vi "FeedbackDecode_UpdateDecodeClustElect.vi"(2 "DecodeClustIn":T1={"TrainParams"={"Lag"=0.0, "KernelWidth"=0.3, "TargRad"=0.15}, "Kinematics"={"Thumb"=0.0, "Index"=0.0, "Middle"=0.0, "Ring"=0.0, "Little"=0.0, "ThumbInt"=0.0, "IndexInt"=0.0, "RingInt"=0.0, "LittleInt"=0.0, "Wrist"=0.0, "WristYaw"=0.0, "WristRoll"=0.0}, "CtrlButtons"={"AcqTraining"=FALSE, "ApplyBaseline"=FALSE, "ApplyTraining"=FALSE, "LoadTrainFile"=FALSE, "CAR"=FALSE, "NIPSpikes"=FALSE, "AcqBaseline"=FALSE, "Stop"=FALSE, "ResetTrial"=FALSE, "CalDEKA"=FALSE, "HideSphrs"=FALSE, "StartTrials"=FALSE, "AutoPop"=FALSE, "ResetVRE"=FALSE, "StopVRE"=FALSE, "AcqCAR"=FALSE, "ConARD"=FALSE, "DEKARestart"=FALSE, "ConnDEKA"=FALSE}, "CompID"={"LV"={"Name"="PNILABVIEW", "IP"="155.100.90.215"}, "ML"={"Name"="PNIMATLAB", "IP"="155.100.91.231"}}, "KMvntClust"={"KGain"=[[1.0, 1.0, -1.0, 1.0], [1.0, 1.0, -1.0, 1.0], [1.0, 1.0, -1.0, 1.0], [1.0, 1.0, -1.0, 1.0], [1.0, 1.0, -1.0, 1.0], [1.0, 1.0, -1.0, 1.0], [1.0, 1.0, -1.0, 1.0], [1.0, 1.0, -1.0, 1.0], [1.0, 1.0, -1.0, 1.0], [1.0, 1.0, -1.0, 1.0], [1.0, 1.0, -1.0, 1.0], [1.0, 1.0, -1.0, 1.0]], "KMvnts"={"Thumb"=FALSE, "Index"=FALSE, "Middle"=FALSE, "Ring"=FALSE, "Little"=FALSE, "ThumbInt"=FALSE, "IndexInt"=FALSE, "RingInt"=FALSE, "LittleInt"=FALSE, "WristPitch"=FALSE, "WristYaw"=FALSE, "WristRoll"=FALSE}, "KThresh"=[[0.2, 0.2, -1.0, 1.0], [0.2, 0.2, -1.0, 1.0], [0.2, 0.2, -1.0, 1.0], [0.2, 0.2, -1.0, 1.0], [0.2, 0.2, -1.0, 1.0], [0.2, 0.2, -1.0, 1.0], [0.2, 0.2, -1.0, 1.0], [0.2, 0.2, -1.0, 1.0], [0.2, 0.2, -1.0, 1.0], [0.2, 0.2, -1.0, 1.0], [0.2, 0.2, -1.0, 1.0], [0.2, 0.2, -1.0, 1.0]], "CtrlMode"=[], "CtrlSpd"=[]}, "ClearUEA"=FALSE, "Targets"={"Thumb"=0.0, "Index"=0.0, "Middle"=0.0, "Ring"=0.0, "Little"=0.0, "ThumbInt"=0.0, "IndexInt"=0.0, "RingInt"=0.0, "LittleInt"=0.0, "Wrist"=0.0, "WristYaw"=0.0, "WristRoll"=0.0}, "KUEAArray"=[{"Boolean 1"=FALSE, "Boolean 2"=FALSE, "Boolean 3"=FALSE, "Boolean 4"=FALSE, "Boolean 5"=FALSE, "Boolean 6"=FALSE, "Boolean 7"=FALSE, "Boolean 8"=FALSE, "Boolean 9"=FALSE, "Boolean 10"=FALSE, "Boolean 11"=FALSE, "Boolean 12"=FALSE, "Boolean 13"=FALSE, "Boolean 14"=FALSE, "Boolean 15"=FALSE, "Boolean 16"=FALSE, "Boolean 17"=FALSE, "Boolean 18"=FALSE, "Boolean 19"=FALSE, "Boolean 20"=FALSE, "Boolean 21"=FALSE, "Boolean 22"=FALSE, "Boolean 23"=FALSE, "Boolean 24"=FALSE, "Boolean 25"=FALSE, "Boolean 26"=FALSE, "Boolean 27"=FALSE, "Boolean 28"=FALSE, "Boolean 29"=FALSE, "Boolean 30"=FALSE, "Boolean 31"=FALSE, "Boolean 32"=FALSE, "Boolean 33"=FALSE, "Boolean 34"=FALSE, "Boolean 35"=FALSE, "Boolean 36"=FALSE, "Boolean 37"=FALSE, "Boolean 38"=FALSE, "Boolean 39"=FALSE, "Boolean 40"=FALSE, "Boolean 41"=FALSE, "Boolean 42"=FALSE, "Boolean 43"=FALSE, "Boolean 44"=FALSE, "Boolean 45"=FALSE, "Boolean 46"=FALSE, "Boolean 47"=FALSE, "Boolean 48"=FALSE, "Boolean 49"=FALSE, "Boolean 50"=FALSE, "Boolean 51"=FALSE, "Boolean 52"=FALSE, "Boolean 53"=FALSE, "Boolean 54"=FALSE, "Boolean 55"=FALSE, "Boolean 56"=FALSE, "Boolean 57"=FALSE, "Boolean 58"=FALSE, "Boolean 59"=FALSE, "Boolean 60"=FALSE, "Boolean 61"=FALSE, "Boolean 62"=FALSE, "Boolean 63"=FALSE, "Boolean 64"=FALSE, "Boolean 65"=FALSE, "Boolean 66"=FALSE, "Boolean 67"=FALSE, "Boolean 68"=FALSE, "Boolean 69"=FALSE, "Boolean 70"=FALSE, "Boolean 71"=FALSE, "Boolean 72"=FALSE, "Boolean 73"=FALSE, "Boolean 74"=FALSE, "Boolean 75"=FALSE, "Boolean 76"=FALSE, "Boolean 77"=FALSE, "Boolean 78"=FALSE, "Boolean 79"=FALSE, "Boolean 80"=FALSE, "Boolean 81"=FALSE, "Boolean 82"=FALSE, "Boolean 83"=FALSE, "Boolean 84"=FALSE, "Boolean 85"=FALSE, "Boolean 86"=FALSE, "Boolean 87"=FALSE, "Boolean 88"=FALSE, "Boolean 89"=FALSE, "Boolean 90"=FALSE, "Boolean 91"=FALSE, "Boolean 92"=FALSE, "Boolean 93"=FALSE, "Boolean 94"=FALSE, "Boolean 95"=FALSE, "Boolean 96"=FALSE, "Boolean 97"=FALSE, "Boolean 98"=FALSE, "Boolean 99"=FALSE, "Boolean 100"=FALSE}, {"Boolean 1"=FALSE, "Boolean 2"=FALSE, "Boolean 3"=FALSE, "Boolean 4"=FALSE, "Boolean 5"=FALSE, "Boolean 6"=FALSE, "Boolean 7"=FALSE, "Boolean 8"=FALSE, "Boolean 9"=FALSE, "Boolean 10"=FALSE, "Boolean 11"=FALSE, "Boolean 12"=FALSE, "Boolean 13"=FALSE, "Boolean 14"=FALSE, "Boolean 15"=FALSE, "Boolean 16"=FALSE, "Boolean 17"=FALSE, "Boolean 18"=FALSE, "Boolean 19"=FALSE, "Boolean 20"=FALSE, "Boolean 21"=FALSE, "Boolean 22"=FALSE, "Boolean 23"=FALSE, "Boolean 24"=FALSE, "Boolean 25"=FALSE, "Boolean 26"=FALSE, "Boolean 27"=FALSE, "Boolean 28"=FALSE, "Boolean 29"=FALSE, "Boolean 30"=FALSE, "Boolean 31"=FALSE, "Boolean 32"=FALSE, "Boolean 33"=FALSE, "Boolean 34"=FALSE, "Boolean 35"=FALSE, "Boolean 36"=FALSE, "Boolean 37"=FALSE, "Boolean 38"=FALSE, "Boolean 39"=FALSE, "Boolean 40"=FALSE, "Boolean 41"=FALSE, "Boolean 42"=FALSE, "Boolean 43"=FALSE, "Boolean 44"=FALSE, "Boolean 45"=FALSE, "Boolean 46"=FALSE, "Boolean 47"=FALSE, "Boolean 48"=FALSE, "Boolean 49"=FALSE, "Boolean 50"=FALSE, "Boolean 51"=FALSE, "Boolean 52"=FALSE, "Boolean 53"=FALSE, "Boolean 54"=FALSE, "Boolean 55"=FALSE, "Boolean 56"=FALSE, "Boolean 57"=FALSE, "Boolean 58"=FALSE, "Boolean 59"=FALSE, "Boolean 60"=FALSE, "Boolean 61"=FALSE, "Boolean 62"=FALSE, "Boolean 63"=FALSE, "Boolean 64"=FALSE, "Boolean 65"=FALSE, "Boolean 66"=FALSE, "Boolean 67"=FALSE, "Boolean 68"=FALSE, "Boolean 69"=FALSE, "Boolean 70"=FALSE, "Boolean 71"=FALSE, "Boolean 72"=FALSE, "Boolean 73"=FALSE, "Boolean 74"=FALSE, "Boolean 75"=FALSE, "Boolean 76"=FALSE, "Boolean 77"=FALSE, "Boolean 78"=FALSE, "Boolean 79"=FALSE, "Boolean 80"=FALSE, "Boolean 81"=FALSE, "Boolean 82"=FALSE, "Boolean 83"=FALSE, "Boolean 84"=FALSE, "Boolean 85"=FALSE, "Boolean 86"=FALSE, "Boolean 87"=FALSE, "Boolean 88"=FALSE, "Boolean 89"=FALSE, "Boolean 90"=FALSE, "Boolean 91"=FALSE, "Boolean 92"=FALSE, "Boolean 93"=FALSE, "Boolean 94"=FALSE, "Boolean 95"=FALSE, "Boolean 96"=FALSE, "Boolean 97"=FALSE, "Boolean 98"=FALSE, "Boolean 99"=FALSE, "Boolean 100"=FALSE}], "ReTrain"=FALSE, "TargDist"=[0.0, 0.0, 0.0, 0.0, 0.0, 0.0], "State"=enum."Initialize", "KalmanType"=enum."Standard", "EventStr"="", "SelElect"=1.0, "KinSrc"=enum."Training", "HoverElect"=0.0, "RasterWin"=1.0, "WfCnt"=15.0, "ClearWfs"=FALSE, "ApplyThresh"=FALSE, "ThreshVal"=-5.0, "ThreshMode"=enum."RMS Single", "DataFolder"="00000000-000000", "ClearEMG"=FALSE, "KEMGClust"={"Boolean 92"=FALSE, "Boolean 82"=FALSE, "Boolean 72"=FALSE, "Boolean 62"=FALSE, "Boolean 52"=FALSE, "Boolean 42"=FALSE, "Boolean 32"=FALSE, "Boolean 22"=FALSE, "Boolean 12"=FALSE, "Boolean 2"=FALSE, "Boolean 93"=FALSE, "Boolean 83"=FALSE, "Boolean 73"=FALSE, "Boolean 63"=FALSE, "Boolean 53"=FALSE, "Boolean 43"=FALSE, "Boolean 33"=FALSE, "Boolean 23"=FALSE, "Boolean 13"=FALSE, "Boolean 3"=FALSE, "Boolean 94"=FALSE, "Boolean 84"=FALSE, "Boolean 74"=FALSE, "Boolean 64"=FALSE, "Boolean 54"=FALSE, "Boolean 44"=FALSE, "Boolean 34"=FALSE, "Boolean 24"=FALSE, "Boolean 14"=FALSE, "Boolean 4"=FALSE, "Boolean 95"=FALSE, "Boolean 85"=FALSE, "Boolean 75"=FALSE, "Boolean 65"=FALSE, "Boolean 55"=FALSE, "Boolean 45"=FALSE, "Boolean 35"=FALSE, "Boolean 25"=FALSE, "Boolean 15"=FALSE, "Boolean 5"=FALSE, "Boolean 96"=FALSE, "Boolean 86"=FALSE, "Boolean 76"=FALSE, "Boolean 66"=FALSE, "Boolean 56"=FALSE, "Boolean 46"=FALSE, "Boolean 36"=FALSE, "Boolean 26"=FALSE, "Boolean 16"=FALSE, "Boolean 6"=FALSE, "Boolean 97"=FALSE, "Boolean 87"=FALSE, "Boolean 77"=FALSE, "Boolean 67"=FALSE, "Boolean 57"=FALSE, "Boolean 47"=FALSE, "Boolean 37"=FALSE, "Boolean 27"=FALSE, "Boolean 17"=FALSE, "Boolean 7"=FALSE, "Boolean 98"=FALSE, "Boolean 88"=FALSE, "Boolean 78"=FALSE, "Boolean 68"=FALSE, "Boolean 58"=FALSE, "Boolean 48"=FALSE, "Boolean 38"=FALSE, "Boolean 28"=FALSE, "Boolean 18"=FALSE, "Boolean 8"=FALSE, "Boolean 99"=FALSE, "Boolean 89"=FALSE, "Boolean 79"=FALSE, "Boolean 69"=FALSE, "Boolean 59"=FALSE, "Boolean 49"=FALSE, "Boolean 39"=FALSE, "Boolean 29"=FALSE, "Boolean 19"=FALSE, "Boolean 9"=FALSE}, "EvntFlag"=FALSE, "FillUEA"=FALSE, "FillEMG"=FALSE, "FillMvnts"=FALSE, "BadUEAElects"=[], "KEMGExtra"=[], "AllPairs"=FALSE, "AutoThresh"=0.4, "BadEMGChans"=[], "LinkedDOF"="{}", "AutoPopType"=enum."Standard", "CARType"=enum."Standard", "*Map"=enum."pNeural/pEMG", "GainFill"=1.0, "ThreshFill"=1.0, "TestType"=enum."MSMS", "Outcome"=enum."---", "TrialCnt"=[], "ClearTrials"=FALSE, "Log10"=FALSE, "KDFFile"="{}", "LimitExt"=FALSE, "*Prosthesis"=enum."MaleLeft", "StartML"=FALSE, "StartMLAux"=FALSE, "StartRec"=FALSE, "DynaThr"=FALSE, "ModeFill"=enum."Position", "SpdFill"=1.0, "DEKAMode"=enum."Velocity", "FreeParam"=0.4, "GoalNoise"=0.4, "Load NN"=FALSE, "ExportTrain"=FALSE, "NumComp"=enum."2 Computers", "DataDir"="00000000-000000", "BuildDir"="00000000-000000", "LatchingFilter"=FALSE, "Trigger"=FALSE, "StartARD"=FALSE, "StartTaska"=FALSE, "StartTaskaSens"=FALSE, "BarBtn"=FALSE} {"SpdFill" min=0.0 max=10.0 step=0.1; "RasterWin" min=1.0 max=30.0 step=1.0; "ThreshFill" min=0.0 max=10.0 step=0.01; "GainFill" min=0.0 max=10.0 step=0.1; "AutoThresh" min=0.0 max=1.0; "Targets"."LittleInt" min=0.0 max=1.0 step=0.01; "Targets"."WristRoll" min=0.0 max=1.0 step=0.01; "Targets"."WristYaw" min=0.0 max=1.0 step=0.01; "Targets"."Wrist" min=0.0 max=1.0 step=0.01; "Targets"."Little" min=0.0 max=1.0 step=0.01; "Targets"."Thumb" min=0.0 max=1.0 step=0.01; "Targets"."RingInt" min=0.0 max=1.0 step=0.01; "Targets"."IndexInt" min=0.0 max=1.0 step=0.01; "Targets"."ThumbInt" min=0.0 max=1.0 step=0.01; "Targets"."Ring" min=0.0 max=1.0 step=0.01; "Targets"."Middle" min=0.0 max=1.0 step=0.01; "Targets"."Index" min=0.0 max=1.0 step=0.01; "KMvntClust"."CtrlSpd" min=0 max=10; "KMvntClust"."KThresh" min=0 max=1; "KMvntClust"."KGain" min=0; "Kinematics"."LittleInt" min=0.0 max=1.0 step=0.01; "Kinematics"."WristRoll" min=0.0 max=1.0 step=0.01; "Kinematics"."WristYaw" min=0.0 max=1.0 step=0.01; "Kinematics"."Wrist" min=0.0 max=1.0 step=0.01; "Kinematics"."Little" min=0.0 max=1.0 step=0.01; "Kinematics"."Thumb" min=0.0 max=1.0 step=0.01; "Kinematics"."RingInt" min=0.0 max=1.0 step=0.01; "Kinematics"."IndexInt" min=0.0 max=1.0 step=0.01; "Kinematics"."ThumbInt" min=0.0 max=1.0 step=0.01; "Kinematics"."Ring" min=0.0 max=1.0 step=0.01; "Kinematics"."Middle" min=0.0 max=1.0 step=0.01; "Kinematics"."Index" min=0.0 max=1.0 step=0.01; "TrainParams"."TargRad" step=0.05 format="%#.2g"; "TrainParams"."KernelWidth" step=0.05 format="%#.2g"}, 3 "KalmanElect":dbl=1.0) -> (0 "DecodeClustOut":T1={"TrainParams"={"Lag"=0.0, "KernelWidth"=0.3, "TargRad"=0.15}, "Kinematics"={"Thumb"=0.0, "Index"=0.0, "Middle"=0.0, "Ring"=0.0, "Little"=0.0, "ThumbInt"=0.0, "IndexInt"=0.0, "RingInt"=0.0, "LittleInt"=0.0, "Wrist"=0.0, "WristYaw"=0.0, "WristRoll"=0.0}, "CtrlButtons"={"AcqTraining"=FALSE, "ApplyBaseline"=FALSE, "ApplyTraining"=FALSE, "LoadTrainFile"=FALSE, "CAR"=FALSE, "NIPSpikes"=FALSE, "AcqBaseline"=FALSE, "Stop"=FALSE, "ResetTrial"=FALSE, "CalDEKA"=FALSE, "HideSphrs"=FALSE, "StartTrials"=FALSE, "AutoPop"=FALSE, "ResetVRE"=FALSE, "StopVRE"=FALSE, "AcqCAR"=FALSE, "ConARD"=FALSE, "DEKARestart"=FALSE, "ConnDEKA"=FALSE}, "CompID"={"LV"={"Name"="PNILABVIEW", "IP"="155.100.90.215"}, "ML"={"Name"="PNIMATLAB", "IP"="155.100.91.231"}}, "KMvntClust"={"KGain"=[[1.0, 1.0, -1.0, 1.0], [1.0, 1.0, -1.0, 1.0], [1.0, 1.0, -1.0, 1.0], [1.0, 1.0, -1.0, 1.0], [1.0, 1.0, -1.0, 1.0], [1.0, 1.0, -1.0, 1.0], [1.0, 1.0, -1.0, 1.0], [1.0, 1.0, -1.0, 1.0], [1.0, 1.0, -1.0, 1.0], [1.0, 1.0, -1.0, 1.0], [1.0, 1.0, -1.0, 1.0], [1.0, 1.0, -1.0, 1.0]], "KMvnts"={"Thumb"=FALSE, "Index"=FALSE, "Middle"=FALSE, "Ring"=FALSE, "Little"=FALSE, "ThumbInt"=FALSE, "IndexInt"=FALSE, "RingInt"=FALSE, "LittleInt"=FALSE, "WristPitch"=FALSE, "WristYaw"=FALSE, "WristRoll"=FALSE}, "KThresh"=[[0.2, 0.2, -1.0, 1.0], [0.2, 0.2, -1.0, 1.0], [0.2, 0.2, -1.0, 1.0], [0.2, 0.2, -1.0, 1.0], [0.2, 0.2, -1.0, 1.0], [0.2, 0.2, -1.0, 1.0], [0.2, 0.2, -1.0, 1.0], [0.2, 0.2, -1.0, 1.0], [0.2, 0.2, -1.0, 1.0], [0.2, 0.2, -1.0, 1.0], [0.2, 0.2, -1.0, 1.0], [0.2, 0.2, -1.0, 1.0]], "CtrlMode"=[], "CtrlSpd"=[]}, "ClearUEA"=FALSE, "Targets"={"Thumb"=0.0, "Index"=0.0, "Middle"=0.0, "Ring"=0.0, "Little"=0.0, "ThumbInt"=0.0, "IndexInt"=0.0, "RingInt"=0.0, "LittleInt"=0.0, "Wrist"=0.0, "WristYaw"=0.0, "WristRoll"=0.0}, "KUEAArray"=[{"Boolean 1"=FALSE, "Boolean 2"=FALSE, "Boolean 3"=FALSE, "Boolean 4"=FALSE, "Boolean 5"=FALSE, "Boolean 6"=FALSE, "Boolean 7"=FALSE, "Boolean 8"=FALSE, "Boolean 9"=FALSE, "Boolean 10"=FALSE, "Boolean 11"=FALSE, "Boolean 12"=FALSE, "Boolean 13"=FALSE, "Boolean 14"=FALSE, "Boolean 15"=FALSE, "Boolean 16"=FALSE, "Boolean 17"=FALSE, "Boolean 18"=FALSE, "Boolean 19"=FALSE, "Boolean 20"=FALSE, "Boolean 21"=FALSE, "Boolean 22"=FALSE, "Boolean 23"=FALSE, "Boolean 24"=FALSE, "Boolean 25"=FALSE, "Boolean 26"=FALSE, "Boolean 27"=FALSE, "Boolean 28"=FALSE, "Boolean 29"=FALSE, "Boolean 30"=FALSE, "Boolean 31"=FALSE, "Boolean 32"=FALSE, "Boolean 33"=FALSE, "Boolean 34"=FALSE, "Boolean 35"=FALSE, "Boolean 36"=FALSE, "Boolean 37"=FALSE, "Boolean 38"=FALSE, "Boolean 39"=FALSE, "Boolean 40"=FALSE, "Boolean 41"=FALSE, "Boolean 42"=FALSE, "Boolean 43"=FALSE, "Boolean 44"=FALSE, "Boolean 45"=FALSE, "Boolean 46"=FALSE, "Boolean 47"=FALSE, "Boolean 48"=FALSE, "Boolean 49"=FALSE, "Boolean 50"=FALSE, "Boolean 51"=FALSE, "Boolean 52"=FALSE, "Boolean 53"=FALSE, "Boolean 54"=FALSE, "Boolean 55"=FALSE, "Boolean 56"=FALSE, "Boolean 57"=FALSE, "Boolean 58"=FALSE, "Boolean 59"=FALSE, "Boolean 60"=FALSE, "Boolean 61"=FALSE, "Boolean 62"=FALSE, "Boolean 63"=FALSE, "Boolean 64"=FALSE, "Boolean 65"=FALSE, "Boolean 66"=FALSE, "Boolean 67"=FALSE, "Boolean 68"=FALSE, "Boolean 69"=FALSE, "Boolean 70"=FALSE, "Boolean 71"=FALSE, "Boolean 72"=FALSE, "Boolean 73"=FALSE, "Boolean 74"=FALSE, "Boolean 75"=FALSE, "Boolean 76"=FALSE, "Boolean 77"=FALSE, "Boolean 78"=FALSE, "Boolean 79"=FALSE, "Boolean 80"=FALSE, "Boolean 81"=FALSE, "Boolean 82"=FALSE, "Boolean 83"=FALSE, "Boolean 84"=FALSE, "Boolean 85"=FALSE, "Boolean 86"=FALSE, "Boolean 87"=FALSE, "Boolean 88"=FALSE, "Boolean 89"=FALSE, "Boolean 90"=FALSE, "Boolean 91"=FALSE, "Boolean 92"=FALSE, "Boolean 93"=FALSE, "Boolean 94"=FALSE, "Boolean 95"=FALSE, "Boolean 96"=FALSE, "Boolean 97"=FALSE, "Boolean 98"=FALSE, "Boolean 99"=FALSE, "Boolean 100"=FALSE}, {"Boolean 1"=FALSE, "Boolean 2"=FALSE, "Boolean 3"=FALSE, "Boolean 4"=FALSE, "Boolean 5"=FALSE, "Boolean 6"=FALSE, "Boolean 7"=FALSE, "Boolean 8"=FALSE, "Boolean 9"=FALSE, "Boolean 10"=FALSE, "Boolean 11"=FALSE, "Boolean 12"=FALSE, "Boolean 13"=FALSE, "Boolean 14"=FALSE, "Boolean 15"=FALSE, "Boolean 16"=FALSE, "Boolean 17"=FALSE, "Boolean 18"=FALSE, "Boolean 19"=FALSE, "Boolean 20"=FALSE, "Boolean 21"=FALSE, "Boolean 22"=FALSE, "Boolean 23"=FALSE, "Boolean 24"=FALSE, "Boolean 25"=FALSE, "Boolean 26"=FALSE, "Boolean 27"=FALSE, "Boolean 28"=FALSE, "Boolean 29"=FALSE, "Boolean 30"=FALSE, "Boolean 31"=FALSE, "Boolean 32"=FALSE, "Boolean 33"=FALSE, "Boolean 34"=FALSE, "Boolean 35"=FALSE, "Boolean 36"=FALSE, "Boolean 37"=FALSE, "Boolean 38"=FALSE, "Boolean 39"=FALSE, "Boolean 40"=FALSE, "Boolean 41"=FALSE, "Boolean 42"=FALSE, "Boolean 43"=FALSE, "Boolean 44"=FALSE, "Boolean 45"=FALSE, "Boolean 46"=FALSE, "Boolean 47"=FALSE, "Boolean 48"=FALSE, "Boolean 49"=FALSE, "Boolean 50"=FALSE, "Boolean 51"=FALSE, "Boolean 52"=FALSE, "Boolean 53"=FALSE, "Boolean 54"=FALSE, "Boolean 55"=FALSE, "Boolean 56"=FALSE, "Boolean 57"=FALSE, "Boolean 58"=FALSE, "Boolean 59"=FALSE, "Boolean 60"=FALSE, "Boolean 61"=FALSE, "Boolean 62"=FALSE, "Boolean 63"=FALSE, "Boolean 64"=FALSE, "Boolean 65"=FALSE, "Boolean 66"=FALSE, "Boolean 67"=FALSE, "Boolean 68"=FALSE, "Boolean 69"=FALSE, "Boolean 70"=FALSE, "Boolean 71"=FALSE, "Boolean 72"=FALSE, "Boolean 73"=FALSE, "Boolean 74"=FALSE, "Boolean 75"=FALSE, "Boolean 76"=FALSE, "Boolean 77"=FALSE, "Boolean 78"=FALSE, "Boolean 79"=FALSE, "Boolean 80"=FALSE, "Boolean 81"=FALSE, "Boolean 82"=FALSE, "Boolean 83"=FALSE, "Boolean 84"=FALSE, "Boolean 85"=FALSE, "Boolean 86"=FALSE, "Boolean 87"=FALSE, "Boolean 88"=FALSE, "Boolean 89"=FALSE, "Boolean 90"=FALSE, "Boolean 91"=FALSE, "Boolean 92"=FALSE, "Boolean 93"=FALSE, "Boolean 94"=FALSE, "Boolean 95"=FALSE, "Boolean 96"=FALSE, "Boolean 97"=FALSE, "Boolean 98"=FALSE, "Boolean 99"=FALSE, "Boolean 100"=FALSE}], "ReTrain"=FALSE, "TargDist"=[0.0, 0.0, 0.0, 0.0, 0.0, 0.0], "State"=enum."Initialize", "KalmanType"=enum."Standard", "EventStr"="", "SelElect"=1.0, "KinSrc"=enum."Training", "HoverElect"=0.0, "RasterWin"=1.0, "WfCnt"=15.0, "ClearWfs"=FALSE, "ApplyThresh"=FALSE, "ThreshVal"=-5.0, "ThreshMode"=enum."RMS Single", "DataFolder"="00000000-000000", "ClearEMG"=FALSE, "KEMGClust"={"Boolean 92"=FALSE, "Boolean 82"=FALSE, "Boolean 72"=FALSE, "Boolean 62"=FALSE, "Boolean 52"=FALSE, "Boolean 42"=FALSE, "Boolean 32"=FALSE, "Boolean 22"=FALSE, "Boolean 12"=FALSE, "Boolean 2"=FALSE, "Boolean 93"=FALSE, "Boolean 83"=FALSE, "Boolean 73"=FALSE, "Boolean 63"=FALSE, "Boolean 53"=FALSE, "Boolean 43"=FALSE, "Boolean 33"=FALSE, "Boolean 23"=FALSE, "Boolean 13"=FALSE, "Boolean 3"=FALSE, "Boolean 94"=FALSE, "Boolean 84"=FALSE, "Boolean 74"=FALSE, "Boolean 64"=FALSE, "Boolean 54"=FALSE, "Boolean 44"=FALSE, "Boolean 34"=FALSE, "Boolean 24"=FALSE, "Boolean 14"=FALSE, "Boolean 4"=FALSE, "Boolean 95"=FALSE, "Boolean 85"=FALSE, "Boolean 75"=FALSE, "Boolean 65"=FALSE, "Boolean 55"=FALSE, "Boolean 45"=FALSE, "Boolean 35"=FALSE, "Boolean 25"=FALSE, "Boolean 15"=FALSE, "Boolean 5"=FALSE, "Boolean 96"=FALSE, "Boolean 86"=FALSE, "Boolean 76"=FALSE, "Boolean 66"=FALSE, "Boolean 56"=FALSE, "Boolean 46"=FALSE, "Boolean 36"=FALSE, "Boolean 26"=FALSE, "Boolean 16"=FALSE, "Boolean 6"=FALSE, "Boolean 97"=FALSE, "Boolean 87"=FALSE, "Boolean 77"=FALSE, "Boolean 67"=FALSE, "Boolean 57"=FALSE, "Boolean 47"=FALSE, "Boolean 37"=FALSE, "Boolean 27"=FALSE, "Boolean 17"=FALSE, "Boolean 7"=FALSE, "Boolean 98"=FALSE, "Boolean 88"=FALSE, "Boolean 78"=FALSE, "Boolean 68"=FALSE, "Boolean 58"=FALSE, "Boolean 48"=FALSE, "Boolean 38"=FALSE, "Boolean 28"=FALSE, "Boolean 18"=FALSE, "Boolean 8"=FALSE, "Boolean 99"=FALSE, "Boolean 89"=FALSE, "Boolean 79"=FALSE, "Boolean 69"=FALSE, "Boolean 59"=FALSE, "Boolean 49"=FALSE, "Boolean 39"=FALSE, "Boolean 29"=FALSE, "Boolean 19"=FALSE, "Boolean 9"=FALSE}, "EvntFlag"=FALSE, "FillUEA"=FALSE, "FillEMG"=FALSE, "FillMvnts"=FALSE, "BadUEAElects"=[], "KEMGExtra"=[], "AllPairs"=FALSE, "AutoThresh"=0.4, "BadEMGChans"=[], "LinkedDOF"="{}", "AutoPopType"=enum."Standard", "CARType"=enum."Standard", "*Map"=enum."pNeural/pEMG", "GainFill"=1.0, "ThreshFill"=1.0, "TestType"=enum."MSMS", "Outcome"=enum."---", "TrialCnt"=[], "ClearTrials"=FALSE, "Log10"=FALSE, "KDFFile"="{}", "LimitExt"=FALSE, "*Prosthesis"=enum."MaleLeft", "StartML"=FALSE, "StartMLAux"=FALSE, "StartRec"=FALSE, "DynaThr"=FALSE, "ModeFill"=enum."Position", "SpdFill"=1.0, "DEKAMode"=enum."Velocity", "FreeParam"=0.4, "GoalNoise"=0.4, "Load NN"=FALSE, "ExportTrain"=FALSE, "NumComp"=enum."2 Computers", "DataDir"="00000000-000000", "BuildDir"="00000000-000000", "LatchingFilter"=FALSE, "Trigger"=FALSE, "StartARD"=FALSE, "StartTaska"=FALSE, "StartTaskaSens"=FALSE, "BarBtn"=FALSE} {"SpdFill" min=0.0 max=10.0 step=0.1; "RasterWin" min=1.0 max=30.0 step=1.0; "ThreshFill" min=0.0 max=10.0 step=0.01; "GainFill" min=0.0 max=10.0 step=0.1; "AutoThresh" min=0.0 max=1.0; "Targets"."LittleInt" min=0.0 max=1.0 step=0.01; "Targets"."WristRoll" min=0.0 max=1.0 step=0.01; "Targets"."WristYaw" min=0.0 max=1.0 step=0.01; "Targets"."Wrist" min=0.0 max=1.0 step=0.01; "Targets"."Little" min=0.0 max=1.0 step=0.01; "Targets"."Thumb" min=0.0 max=1.0 step=0.01; "Targets"."RingInt" min=0.0 max=1.0 step=0.01; "Targets"."IndexInt" min=0.0 max=1.0 step=0.01; "Targets"."ThumbInt" min=0.0 max=1.0 step=0.01; "Targets"."Ring" min=0.0 max=1.0 step=0.01; "Targets"."Middle" min=0.0 max=1.0 step=0.01; "Targets"."Index" min=0.0 max=1.0 step=0.01; "KMvntClust"."CtrlSpd" min=0 max=10; "KMvntClust"."KThresh" min=0 max=1; "KMvntClust"."KGain" min=0; "Kinematics"."LittleInt" min=0.0 max=1.0 step=0.01; "Kinematics"."WristRoll" min=0.0 max=1.0 step=0.01; "Kinematics"."WristYaw" min=0.0 max=1.0 step=0.01; "Kinematics"."Wrist" min=0.0 max=1.0 step=0.01; "Kinematics"."Little" min=0.0 max=1.0 step=0.01; "Kinematics"."Thumb" min=0.0 max=1.0 step=0.01; "Kinematics"."RingInt" min=0.0 max=1.0 step=0.01; "Kinematics"."IndexInt" min=0.0 max=1.0 step=0.01; "Kinematics"."ThumbInt" min=0.0 max=1.0 step=0.01; "Kinematics"."Ring" min=0.0 max=1.0 step=0.01; "Kinematics"."Middle" min=0.0 max=1.0 step=0.01; "Kinematics"."Index" min=0.0 max=1.0 step=0.01; "TrainParams"."TargRad" step=0.05 format="%#.2g"; "TrainParams"."KernelWidth" step=0.05 format="%#.2g"})   [LabVIEW 2020]
uses:
  FeedbackDecode_DecodeClust.ctl
panel:
  # "G"
  # "T"
  # "Mode"
  # "S"
  # "Negative lag shifts feature variables left (earlier)"
  # "{[1,2,4];[5,3];[6,7,8]}"
  # "Select before apply training"
  # "1"
  # "2"
  # "3"
  # "4"
  # "5"
  # "6"
  # "7"
  # "8"
  # "1"
  # "2"
  # "3"
  # "4"
  # "1-2"
  # "1-3"
  # "1-4"
  # "2-3"
  # "2-4"
  # "3-4"
  # "DOF"
  # "Gain (F/E)"
  # "Thresh (F/E)"
  # "Mode"
  # "Spd"
  # "G"
  # "T"
  # "Mode"
  # "S"
  # "Negative lag shifts feature variables left (earlier)"
  # "{[1,2,4];[5,3];[6,7,8]}"
  # "Select before apply training"
  # "1"
  # "2"
  # "3"
  # "4"
  # "5"
  # "6"
  # "7"
  # "8"
  # "1"
  # "2"
  # "3"
  # "4"
  # "1-2"
  # "1-3"
  # "1-4"
  # "2-3"
  # "2-4"
  # "3-4"
  # "DOF"
  # "Gain (F/E)"
  # "Thresh (F/E)"
  # "Mode"
  # "Spd"
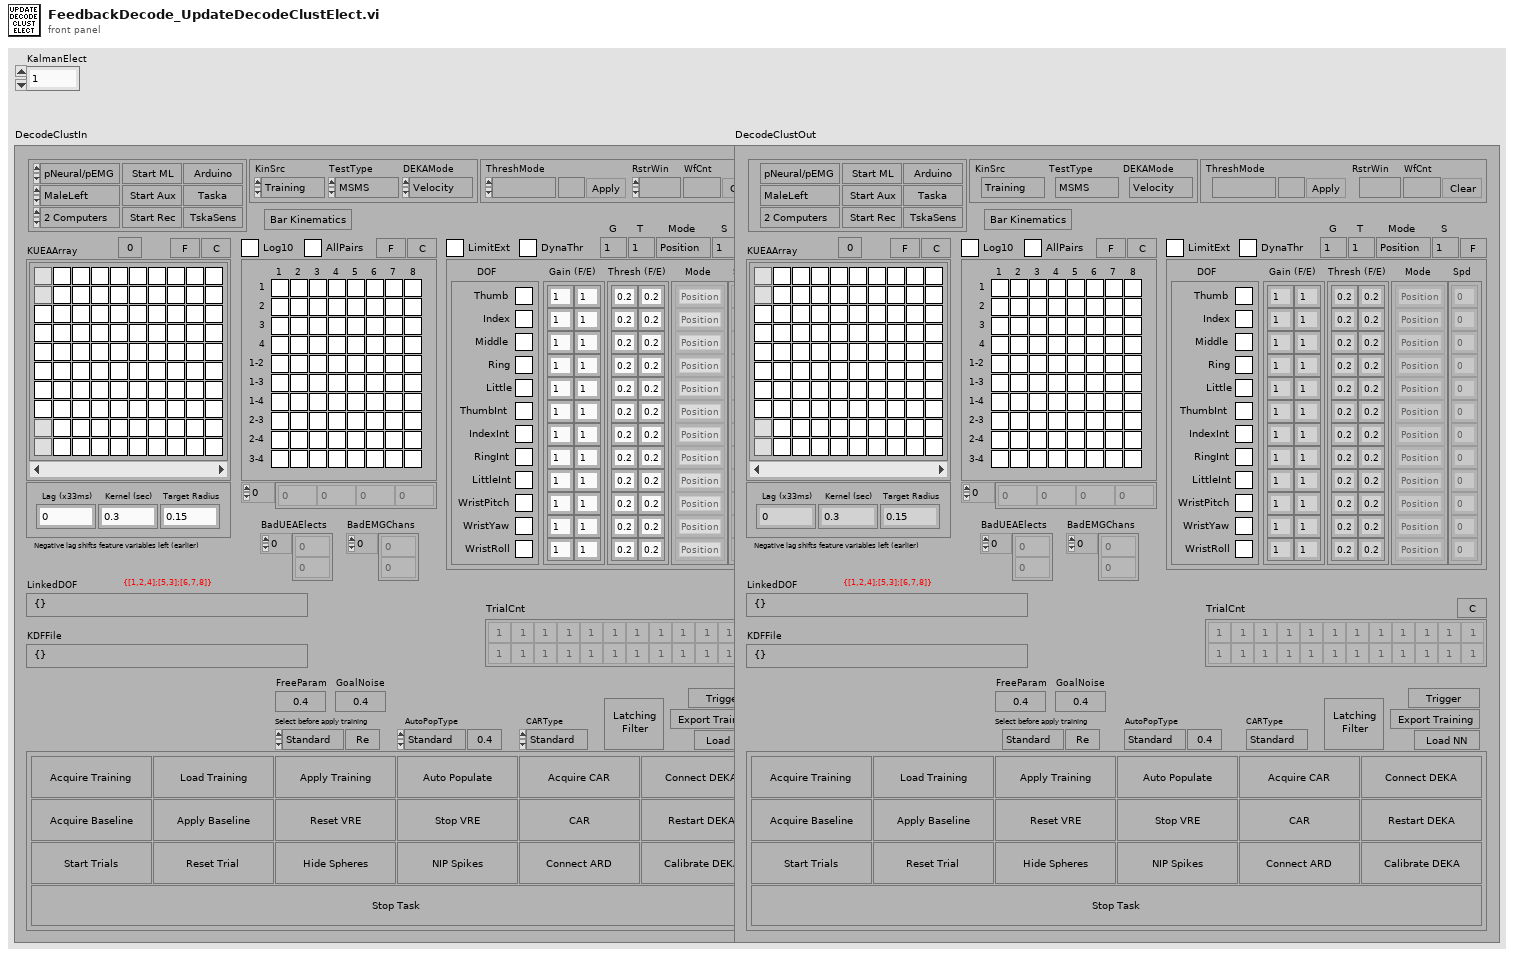
[diagram p1: front panel]
types:
  T1 = typedef "FeedbackDecode_DecodeClust.ctl" = cluster{"TrainParams":cluster{"Lag":dbl, "KernelWidth":dbl, "TargRad":dbl}, "Kinematics":cluster{"Thumb":dbl, "Index":dbl, "Middle":dbl, "Ring":dbl, "Little":dbl, "ThumbInt":dbl, "IndexInt":dbl, "RingInt":dbl, "LittleInt":dbl, "Wrist":dbl, "WristYaw":dbl, "WristRoll":dbl}, "CtrlButtons":cluster{"AcqTraining":bool, "ApplyBaseline":bool, "ApplyTraining":bool, "LoadTrainFile":bool, "CAR":bool, "NIPSpikes":bool, "AcqBaseline":bool, "Stop":bool, "ResetTrial":bool, "CalDEKA":bool, "HideSphrs":bool, "StartTrials":bool, "AutoPop":bool, "ResetVRE":bool, "StopVRE":bool, "AcqCAR":bool, "ConARD":bool, "DEKARestart":bool, "ConnDEKA":bool}, "CompID":cluster{"LV":cluster{"Name":string, "IP":string}, "ML":cluster{"Name":string, "IP":string}}, "KMvntClust":cluster{"KGain":sgl[][], "KMvnts":cluster{"Thumb":bool, "Index":bool, "Middle":bool, "Ring":bool, "Little":bool, "ThumbInt":bool, "IndexInt":bool, "RingInt":bool, "LittleInt":bool, "WristPitch":bool, "WristYaw":bool, "WristRoll":bool}, "KThresh":sgl[][], "CtrlMode":enum16{"Position", "Latching", "Leaky", "Velocity"}[], "CtrlSpd":sgl[]}, "ClearUEA":bool, "Targets":cluster{"Thumb":dbl, "Index":dbl, "Middle":dbl, "Ring":dbl, "Little":dbl, "ThumbInt":dbl, "IndexInt":dbl, "RingInt":dbl, "LittleInt":dbl, "Wrist":dbl, "WristYaw":dbl, "WristRoll":dbl}, "KUEAArray":cluster{"Boolean 1":bool, "Boolean 2":bool, "Boolean 3":bool, "Boolean 4":bool, "Boolean 5":bool, "Boolean 6":bool, "Boolean 7":bool, "Boolean 8":bool, "Boolean 9":bool, "Boolean 10":bool, "Boolean 11":bool, "Boolean 12":bool, "Boolean 13":bool, "Boolean 14":bool, "Boolean 15":bool, "Boolean 16":bool, "Boolean 17":bool, "Boolean 18":bool, "Boolean 19":bool, "Boolean 20":bool, "Boolean 21":bool, "Boolean 22":bool, "Boolean 23":bool, "Boolean 24":bool, "Boolean 25":bool, "Boolean 26":bool, "Boolean 27":bool, "Boolean 28":bool, "Boolean 29":bool, "Boolean 30":bool, "Boolean 31":bool, "Boolean 32":bool, "Boolean 33":bool, "Boolean 34":bool, "Boolean 35":bool, "Boolean 36":bool, "Boolean 37":bool, "Boolean 38":bool, "Boolean 39":bool, "Boolean 40":bool, "Boolean 41":bool, "Boolean 42":bool, "Boolean 43":bool, "Boolean 44":bool, "Boolean 45":bool, "Boolean 46":bool, "Boolean 47":bool, "Boolean 48":bool, "Boolean 49":bool, "Boolean 50":bool, "Boolean 51":bool, "Boolean 52":bool, "Boolean 53":bool, "Boolean 54":bool, "Boolean 55":bool, "Boolean 56":bool, "Boolean 57":bool, "Boolean 58":bool, "Boolean 59":bool, "Boolean 60":bool, "Boolean 61":bool, "Boolean 62":bool, "Boolean 63":bool, "Boolean 64":bool, "Boolean 65":bool, "Boolean 66":bool, "Boolean 67":bool, "Boolean 68":bool, "Boolean 69":bool, "Boolean 70":bool, "Boolean 71":bool, "Boolean 72":bool, "Boolean 73":bool, "Boolean 74":bool, "Boolean 75":bool, "Boolean 76":bool, "Boolean 77":bool, "Boolean 78":bool, "Boolean 79":bool, "Boolean 80":bool, "Boolean 81":bool, "Boolean 82":bool, "Boolean 83":bool, "Boolean 84":bool, "Boolean 85":bool, "Boolean 86":bool, "Boolean 87":bool, "Boolean 88":bool, "Boolean 89":bool, "Boolean 90":bool, "Boolean 91":bool, "Boolean 92":bool, "Boolean 93":bool, "Boolean 94":bool, "Boolean 95":bool, "Boolean 96":bool, "Boolean 97":bool, "Boolean 98":bool, "Boolean 99":bool, "Boolean 100":bool}[], "ReTrain":bool, "TargDist":dbl[], "State":enum16{"Initialize", "Acquire Start", "Acquire Response", "Finalize"}, "KalmanType":enum16{"Standard", "Mean", "Refit", "LinSVReg", "NonLinSVReg", "PCA", "DWPRR", "AdaptKF", "NN", "NN_python", "AdaptKF2", "KF_Short_Goal"}, "EventStr":string, "SelElect":dbl, "KinSrc":enum16{"Off", "Training", "Decode", "COB", "LEAP"}, "HoverElect":dbl, "RasterWin":dbl, "WfCnt":dbl, "ClearWfs":bool, "ApplyThresh":bool, "ThreshVal":dbl, "ThreshMode":enum16{"RMS Single", "RMS All", "RMS Auto", "Volt Single", "Volt All"}, "DataFolder":string, "ClearEMG":bool, "KEMGClust":cluster{"Boolean 92":bool, "Boolean 82":bool, "Boolean 72":bool, "Boolean 62":bool, "Boolean 52":bool, "Boolean 42":bool, "Boolean 32":bool, "Boolean 22":bool, "Boolean 12":bool, "Boolean 2":bool, "Boolean 93":bool, "Boolean 83":bool, "Boolean 73":bool, "Boolean 63":bool, "Boolean 53":bool, "Boolean 43":bool, "Boolean 33":bool, "Boolean 23":bool, "Boolean 13":bool, "Boolean 3":bool, "Boolean 94":bool, "Boolean 84":bool, "Boolean 74":bool, "Boolean 64":bool, "Boolean 54":bool, "Boolean 44":bool, "Boolean 34":bool, "Boolean 24":bool, "Boolean 14":bool, "Boolean 4":bool, "Boolean 95":bool, "Boolean 85":bool, "Boolean 75":bool, "Boolean 65":bool, "Boolean 55":bool, "Boolean 45":bool, "Boolean 35":bool, "Boolean 25":bool, "Boolean 15":bool, "Boolean 5":bool, "Boolean 96":bool, "Boolean 86":bool, "Boolean 76":bool, "Boolean 66":bool, "Boolean 56":bool, "Boolean 46":bool, "Boolean 36":bool, "Boolean 26":bool, "Boolean 16":bool, "Boolean 6":bool, "Boolean 97":bool, "Boolean 87":bool, "Boolean 77":bool, "Boolean 67":bool, "Boolean 57":bool, "Boolean 47":bool, "Boolean 37":bool, "Boolean 27":bool, "Boolean 17":bool, "Boolean 7":bool, "Boolean 98":bool, "Boolean 88":bool, "Boolean 78":bool, "Boolean 68":bool, "Boolean 58":bool, "Boolean 48":bool, "Boolean 38":bool, "Boolean 28":bool, "Boolean 18":bool, "Boolean 8":bool, "Boolean 99":bool, "Boolean 89":bool, "Boolean 79":bool, "Boolean 69":bool, "Boolean 59":bool, "Boolean 49":bool, "Boolean 39":bool, "Boolean 29":bool, "Boolean 19":bool, "Boolean 9":bool}, "EvntFlag":bool, "FillUEA":bool, "FillEMG":bool, "FillMvnts":bool, "BadUEAElects":dbl[], "KEMGExtra":dbl[], "AllPairs":bool, "AutoThresh":dbl, "BadEMGChans":dbl[], "LinkedDOF":string, "AutoPopType":enum16{"Standard", "Stepwise", "Gram"}, "CARType":enum16{"Standard", "NN"}, "*Map":enum16{"pNeural/pEMG", "pNeural/aEMG", "aNeural/pEMG", "aNeural/aEMG", "N2021/pEMG"}, "GainFill":dbl, "ThreshFill":dbl, "TestType":enum16{"MSMS", "Bakeoff11", "Bakeoff21", "Bakeoff31", "Bakeoff32", "Bakeoff32_Ball", "Bakeoff32_Checkers", "Bakeoff32_Pen", "FragileBlock"}, "Outcome":enum16{"---", "Success", "Failure"}, "TrialCnt":dbl[][], "ClearTrials":bool, "Log10":bool, "KDFFile":string, "LimitExt":bool, "*Prosthesis":enum16{"MaleRight", "MaleLeft"}, "StartML":bool, "StartMLAux":bool, "StartRec":bool, "DynaThr":bool, "ModeFill":enum16{"Position", "Latching", "Leaky", "Velocity"}, "SpdFill":dbl, "DEKAMode":enum16{"Velocity", "Position"}, "FreeParam":dbl, "GoalNoise":dbl, "Load NN":bool, "ExportTrain":bool, "NumComp":enum16{"1 Computer", "2 Computers"}, "DataDir":string, "BuildDir":string, "LatchingFilter":bool, "Trigger":bool, "StartARD":bool, "StartTaska":bool, "StartTaskaSens":bool, "BarBtn":bool}
  T2 = cluster{"Boolean 92":bool, "Boolean 82":bool, "Boolean 72":bool, "Boolean 62":bool, "Boolean 52":bool, "Boolean 42":bool, "Boolean 32":bool, "Boolean 22":bool, "Boolean 12":bool, "Boolean 2":bool, "Boolean 93":bool, "Boolean 83":bool, "Boolean 73":bool, "Boolean 63":bool, "Boolean 53":bool, "Boolean 43":bool, "Boolean 33":bool, "Boolean 23":bool, "Boolean 13":bool, "Boolean 3":bool, "Boolean 94":bool, "Boolean 84":bool, "Boolean 74":bool, "Boolean 64":bool, "Boolean 54":bool, "Boolean 44":bool, "Boolean 34":bool, "Boolean 24":bool, "Boolean 14":bool, "Boolean 4":bool, "Boolean 95":bool, "Boolean 85":bool, "Boolean 75":bool, "Boolean 65":bool, "Boolean 55":bool, "Boolean 45":bool, "Boolean 35":bool, "Boolean 25":bool, "Boolean 15":bool, "Boolean 5":bool, "Boolean 96":bool, "Boolean 86":bool, "Boolean 76":bool, "Boolean 66":bool, "Boolean 56":bool, "Boolean 46":bool, "Boolean 36":bool, "Boolean 26":bool, "Boolean 16":bool, "Boolean 6":bool, "Boolean 97":bool, "Boolean 87":bool, "Boolean 77":bool, "Boolean 67":bool, "Boolean 57":bool, "Boolean 47":bool, "Boolean 37":bool, "Boolean 27":bool, "Boolean 17":bool, "Boolean 7":bool, "Boolean 98":bool, "Boolean 88":bool, "Boolean 78":bool, "Boolean 68":bool, "Boolean 58":bool, "Boolean 48":bool, "Boolean 38":bool, "Boolean 28":bool, "Boolean 18":bool, "Boolean 8":bool, "Boolean 99":bool, "Boolean 89":bool, "Boolean 79":bool, "Boolean 69":bool, "Boolean 59":bool, "Boolean 49":bool, "Boolean 39":bool, "Boolean 29":bool, "Boolean 19":bool, "Boolean 9":bool}
  T3 = cluster{"KEMGClust[0]":bool, "KEMGClust[1]":bool, "KEMGClust[2]":bool, "KEMGClust[3]":bool, "KEMGClust[4]":bool, "KEMGClust[5]":bool, "KEMGClust[6]":bool, "KEMGClust[7]":bool, "KEMGClust[8]":bool, "KEMGClust[9]":bool, "KEMGClust[10]":bool, "KEMGClust[11]":bool, "KEMGClust[12]":bool, "KEMGClust[13]":bool, "KEMGClust[14]":bool, "KEMGClust[15]":bool, "KEMGClust[16]":bool, "KEMGClust[17]":bool, "KEMGClust[18]":bool, "KEMGClust[19]":bool, "KEMGClust[20]":bool, "KEMGClust[21]":bool, "KEMGClust[22]":bool, "KEMGClust[23]":bool, "KEMGClust[24]":bool, "KEMGClust[25]":bool, "KEMGClust[26]":bool, "KEMGClust[27]":bool, "KEMGClust[28]":bool, "KEMGClust[29]":bool, "KEMGClust[30]":bool, "KEMGClust[31]":bool, "KEMGClust[32]":bool, "KEMGClust[33]":bool, "KEMGClust[34]":bool, "KEMGClust[35]":bool, "KEMGClust[36]":bool, "KEMGClust[37]":bool, "KEMGClust[38]":bool, "KEMGClust[39]":bool, "KEMGClust[40]":bool, "KEMGClust[41]":bool, "KEMGClust[42]":bool, "KEMGClust[43]":bool, "KEMGClust[44]":bool, "KEMGClust[45]":bool, "KEMGClust[46]":bool, "KEMGClust[47]":bool, "KEMGClust[48]":bool, "KEMGClust[49]":bool, "KEMGClust[50]":bool, "KEMGClust[51]":bool, "KEMGClust[52]":bool, "KEMGClust[53]":bool, "KEMGClust[54]":bool, "KEMGClust[55]":bool, "KEMGClust[56]":bool, "KEMGClust[57]":bool, "KEMGClust[58]":bool, "KEMGClust[59]":bool, "KEMGClust[60]":bool, "KEMGClust[61]":bool, "KEMGClust[62]":bool, "KEMGClust[63]":bool, "KEMGClust[64]":bool, "KEMGClust[65]":bool, "KEMGClust[66]":bool, "KEMGClust[67]":bool, "KEMGClust[68]":bool, "KEMGClust[69]":bool, "KEMGClust[70]":bool, "KEMGClust[71]":bool, "KEMGClust[72]":bool, "KEMGClust[73]":bool, "KEMGClust[74]":bool, "KEMGClust[75]":bool, "KEMGClust[76]":bool, "KEMGClust[77]":bool, "KEMGClust[78]":bool, "KEMGClust[79]":bool}
  T4 = cluster{"Boolean 1":bool, "Boolean 2":bool, "Boolean 3":bool, "Boolean 4":bool, "Boolean 5":bool, "Boolean 6":bool, "Boolean 7":bool, "Boolean 8":bool, "Boolean 9":bool, "Boolean 10":bool, "Boolean 11":bool, "Boolean 12":bool, "Boolean 13":bool, "Boolean 14":bool, "Boolean 15":bool, "Boolean 16":bool, "Boolean 17":bool, "Boolean 18":bool, "Boolean 19":bool, "Boolean 20":bool, "Boolean 21":bool, "Boolean 22":bool, "Boolean 23":bool, "Boolean 24":bool, "Boolean 25":bool, "Boolean 26":bool, "Boolean 27":bool, "Boolean 28":bool, "Boolean 29":bool, "Boolean 30":bool, "Boolean 31":bool, "Boolean 32":bool, "Boolean 33":bool, "Boolean 34":bool, "Boolean 35":bool, "Boolean 36":bool, "Boolean 37":bool, "Boolean 38":bool, "Boolean 39":bool, "Boolean 40":bool, "Boolean 41":bool, "Boolean 42":bool, "Boolean 43":bool, "Boolean 44":bool, "Boolean 45":bool, "Boolean 46":bool, "Boolean 47":bool, "Boolean 48":bool, "Boolean 49":bool, "Boolean 50":bool, "Boolean 51":bool, "Boolean 52":bool, "Boolean 53":bool, "Boolean 54":bool, "Boolean 55":bool, "Boolean 56":bool, "Boolean 57":bool, "Boolean 58":bool, "Boolean 59":bool, "Boolean 60":bool, "Boolean 61":bool, "Boolean 62":bool, "Boolean 63":bool, "Boolean 64":bool, "Boolean 65":bool, "Boolean 66":bool, "Boolean 67":bool, "Boolean 68":bool, "Boolean 69":bool, "Boolean 70":bool, "Boolean 71":bool, "Boolean 72":bool, "Boolean 73":bool, "Boolean 74":bool, "Boolean 75":bool, "Boolean 76":bool, "Boolean 77":bool, "Boolean 78":bool, "Boolean 79":bool, "Boolean 80":bool, "Boolean 81":bool, "Boolean 82":bool, "Boolean 83":bool, "Boolean 84":bool, "Boolean 85":bool, "Boolean 86":bool, "Boolean 87":bool, "Boolean 88":bool, "Boolean 89":bool, "Boolean 90":bool, "Boolean 91":bool, "Boolean 92":bool, "Boolean 93":bool, "Boolean 94":bool, "Boolean 95":bool, "Boolean 96":bool, "Boolean 97":bool, "Boolean 98":bool, "Boolean 99":bool, "Boolean 100":bool}[]
  T5 = cluster{"KUEA[0]":bool, "KUEA[1]":bool, "KUEA[2]":bool, "KUEA[3]":bool, "KUEA[4]":bool, "KUEA[5]":bool, "KUEA[6]":bool, "KUEA[7]":bool, "KUEA[8]":bool, "KUEA[9]":bool, "KUEA[10]":bool, "KUEA[11]":bool, "KUEA[12]":bool, "KUEA[13]":bool, "KUEA[14]":bool, "KUEA[15]":bool, "KUEA[16]":bool, "KUEA[17]":bool, "KUEA[18]":bool, "KUEA[19]":bool, "KUEA[20]":bool, "KUEA[21]":bool, "KUEA[22]":bool, "KUEA[23]":bool, "KUEA[24]":bool, "KUEA[25]":bool, "KUEA[26]":bool, "KUEA[27]":bool, "KUEA[28]":bool, "KUEA[29]":bool, "KUEA[30]":bool, "KUEA[31]":bool, "KUEA[32]":bool, "KUEA[33]":bool, "KUEA[34]":bool, "KUEA[35]":bool, "KUEA[36]":bool, "KUEA[37]":bool, "KUEA[38]":bool, "KUEA[39]":bool, "KUEA[40]":bool, "KUEA[41]":bool, "KUEA[42]":bool, "KUEA[43]":bool, "KUEA[44]":bool, "KUEA[45]":bool, "KUEA[46]":bool, "KUEA[47]":bool, "KUEA[48]":bool, "KUEA[49]":bool, "KUEA[50]":bool, "KUEA[51]":bool, "KUEA[52]":bool, "KUEA[53]":bool, "KUEA[54]":bool, "KUEA[55]":bool, "KUEA[56]":bool, "KUEA[57]":bool, "KUEA[58]":bool, "KUEA[59]":bool, "KUEA[60]":bool, "KUEA[61]":bool, "KUEA[62]":bool, "KUEA[63]":bool, "KUEA[64]":bool, "KUEA[65]":bool, "KUEA[66]":bool, "KUEA[67]":bool, "KUEA[68]":bool, "KUEA[69]":bool, "KUEA[70]":bool, "KUEA[71]":bool, "KUEA[72]":bool, "KUEA[73]":bool, "KUEA[74]":bool, "KUEA[75]":bool, "KUEA[76]":bool, "KUEA[77]":bool, "KUEA[78]":bool, "KUEA[79]":bool, "KUEA[80]":bool, "KUEA[81]":bool, "KUEA[82]":bool, "KUEA[83]":bool, "KUEA[84]":bool, "KUEA[85]":bool, "KUEA[86]":bool, "KUEA[87]":bool, "KUEA[88]":bool, "KUEA[89]":bool, "KUEA[90]":bool, "KUEA[91]":bool, "KUEA[92]":bool, "KUEA[93]":bool, "KUEA[94]":bool, "KUEA[95]":bool, "KUEA[96]":bool, "KUEA[97]":bool, "KUEA[98]":bool, "KUEA[99]":bool}
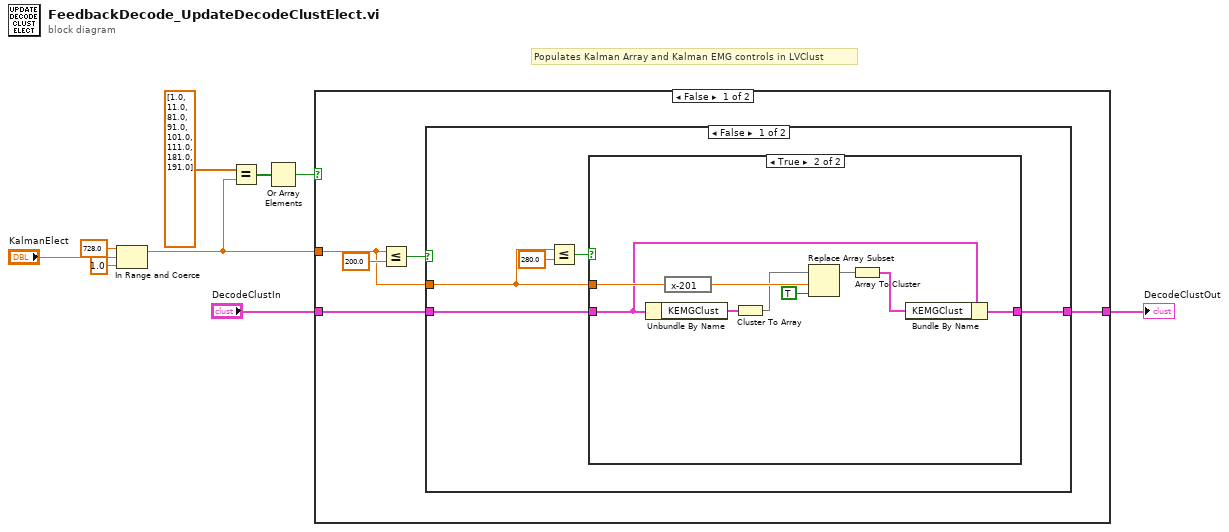
[diagram p0: block diagram]
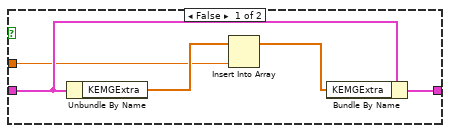
[diagram p2: hidden frame]
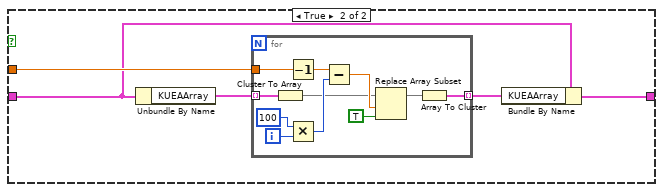
[diagram p3: hidden frame]
diagram:
  # "Populates Kalman Array and Kalman EMG controls in LVClust"
  n1 = In Range and Coerce(upper limit=728.0, x="KalmanElect", lower limit=1.0 ("upper limit")) -> (coerced(x)=w3:dbl)  [unwired: 1 out]
  n2 = Equal?(x=dbl[] [1.0, 11.0, 81.0, 91.0, 101.0, 111.0, 181.0, 191.0], y=w3) -> (x = y?=w8:bool[])
  n3 = Or Array Elements(Boolean array=w8) -> (logical OR=w7:bool)
  n4 = case shown="False" w7 {
    tunnel: "DecodeClustIn" -> [w12 w50]
    tunnel: [w11 w50] -> w1
    tunnel: w3 -> [w10 _]
    frame False {
      n5 = Less Or Equal?(x=w10, y=200.0) -> (x <= y?=w13:bool)
      n6 = case shown="False" w13 {
        tunnel: w10 -> [w17 w38]
        tunnel: w12 -> [w19 w36]
        tunnel: [w18 w34] -> w11
        frame False {
          n7 = Less Or Equal?(x=w17, y=280.0) -> (x <= y?=w15:bool)
          n8 = case shown="True" w15 {
            tunnel: w17 -> [w22 w32]
            tunnel: w19 -> [w24 w27]
            tunnel: [w20 w25] -> w18
            frame False {
              n9 = Unbundle By Name(w24) -> ("KEMGExtra"=w23:dbl[])
              n10 = Insert Into Array(array=w23, new element=w22) -> (w21:dbl[])  [unwired: 1 in]
              n11 = Bundle By Name(cluster=w24, "KEMGExtra"=w21) -> (w20:T1)
            }
            frame True {
              n12 = Unbundle By Name(w27) -> ("KEMGClust"=w33:T2)
              n13 = expression code="x-201"(w32) -> (w29:dbl)
              n14 = Cluster To Array(cluster=w33) -> (array=w28:bool[])
              n15 = Replace Array Subset(array=w28, new element=TRUE ("new element/subarray"), index=w29) -> (w31:bool[])
              n16 = Array To Cluster(array=w31) -> (cluster=w26:T3)
              n17 = Bundle By Name(cluster=w27, "KEMGClust"=w26) -> (w25:T1)
            }
          }
        }
        frame True {
          n18 = Unbundle By Name(w36) -> ("KUEAArray"=w37:T4)
          n19 = for {
            tunnel: w38 -> [w48]
            tunnel: [w47] -> w35 mode=indexing
            tunnel: w37 -> [w40] mode=indexing
            i -> [w46]
            n20 = Cluster To Array(cluster=w40) -> (array=w39:bool[])
            n21 = Decrement(x=w48) -> (x-1=w42:dbl)
            n22 = Multiply(x=100, y=w46) -> (x*y=w44:i32)
            n23 = Subtract(x=w42, y=w44) -> (x-y=w41:dbl)
            n24 = Replace Array Subset(array=w39, new element=TRUE ("new element/subarray"), index=w41) -> (w49:bool[])
            n25 = Array To Cluster(array=w49) -> (cluster=w47:T5)
          }
          n26 = Bundle By Name(cluster=w36, "KUEAArray"=w35) -> (w34:T1)
        }
      }
    }
    frame True {
    }
  }
  "DecodeClustOut" <- w1
